vi "FPGAMain.vi"() -> ()   [LabVIEW 2022 SP3]
uses:
  <vilib>/rvi/Emulation/niFpgaGetClockAttributes.vi
  <vilib>/rvi/Emulation/niFpgaSctlEmulationGetInTimedLoop.vi
  <vilib>/rvi/Emulation/niFpgaEmulationReportErrorSimple.vi
  <vilib>/rvi/interface/RandomDataEmulation/niFpgaRandomDataHandleErrors.vi
  <vilib>/rvi/Emulation/niFpgaEmulationIsFPGAContextNoSignature.vi
  <vilib>/rvi/DataTransferAndStorage/Container/Common/niFpgaContainerGetUniqueNameForEmu.vi
  <vilib>/rvi/Memory/Memory_Emulation/niFpgaMemoryEmulationCacheClearOnFirstRun.vi
  <vilib>/rvi/Memory/Memory_Emulation/nirvimemoryEmulationManagerCache_MakeExclusive.vi
  <vilib>/rvi/Memory/Memory_Emulation/niFpgaMemoryEmulationValidateCache.vi
  <vilib>/rvi/Memory/Memory_Emulation/nirvimemoryEmulationManagerCache_InsertValue.vi
  <vilib>/Utility/error.llb/Clear Errors.vi
  <vilib>/rvi/Memory/Memory_Emulation/nirvimemoryEmulationManagerCache_ReleaseExclusive.vi
  <vilib>/rvi/Memory/Memory_Emulation/nirvimemoryEmulationManagerCache_GetValue.vi
  <vilib>/rvi/Memory/Memory_Emulation/nirvimemoryEmulationManagerCache_SetValue.vi
  <vilib>/rvi/Emulation/niFpgaProcessEmulError.vi
  <vilib>/rvi/DataTransferAndStorage/Container/Common/niFpgaContainerExecOnDevCompGetState.vi
  <vilib>/rvi/errors/niFpgaSetErrorForExecOnDevCompSimple.vi
  <vilib>/rvi/eio/common/nirviEmuReportErrorAndStop.vi
  <vilib>/rvi/FIFO/Fifo_Resource/nirvififoEmulationSetSize.vi
  <vilib>/rvi/FIFO/Fifo_Resource/nirviFifoEmulationQueueMgr.vi
  <instcachedir>/0/nirviFifoEmulationQueueMgr_E5CAEC123FF24DC58D834DCA3CDAA9B5.lvgen/nirviFifoEmulationQueueMgr_E5CAEC123FF24DC58D834DCA3CDAA9B5_005.vi
  <vilib>/rvi/FIFO/Fifo_Resource/nirvififoEmulationDetermineInputValidOut.vi
  <vilib>/rvi/FIFO/Fifo_Resource/nirvififoEmulationCreateLock.vi
  <vilib>/rvi/FIFO/Fifo_Resource/nirvififoEmulationObtainLock.vi
  <vilib>/rvi/FIFO/Fifo_Resource/nirvififoEmulationReleaseLock.vi
  <vilib>/rvi/occurrence/nirviWaitOnOccurrenceBase.vi
  <vilib>/rvi/errors/nirviReportUnexpectedCaseInternalError.vi
  <vilib>/rvi/errors/nirviReportUnexpectedCaseInternalError (U32).vi
  <vilib>/rvi/Emulation/niFpgaCriticalErrorInLSC.vi
  <vilib>/rvi/eio/common/nirviEmuTemplateMethod_errors.vi
  <vilib>/rvi/DataTransferAndStorage/Container/XNode/niFpgaContainer.xnode
  <vilib>/rvi/interface/RandomDataEmulation/nirviRandomDataFpgaReadWriteTemplate.vi
  <vilib>/rvi/DataTransferAndStorage/Register/Emulation/niFpgaRegisterEmulation.vi
  <vilib>/rvi/FIFO/Fifo_Resource/niFpgaFifoEmulationRefIn.vi
  <vilib>/eio/EIONode/EIONode.xnode
panel:
  out "Control Signals":bool[](array[boolean])
  out "Tick Count(uSec)":u16
  out "Mod1/AI0":fxp<+/-,26,5>
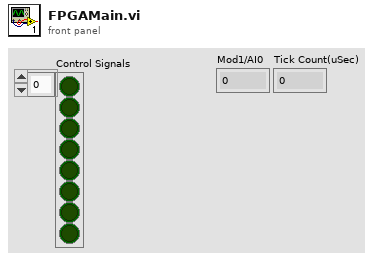
[diagram p1: front panel]
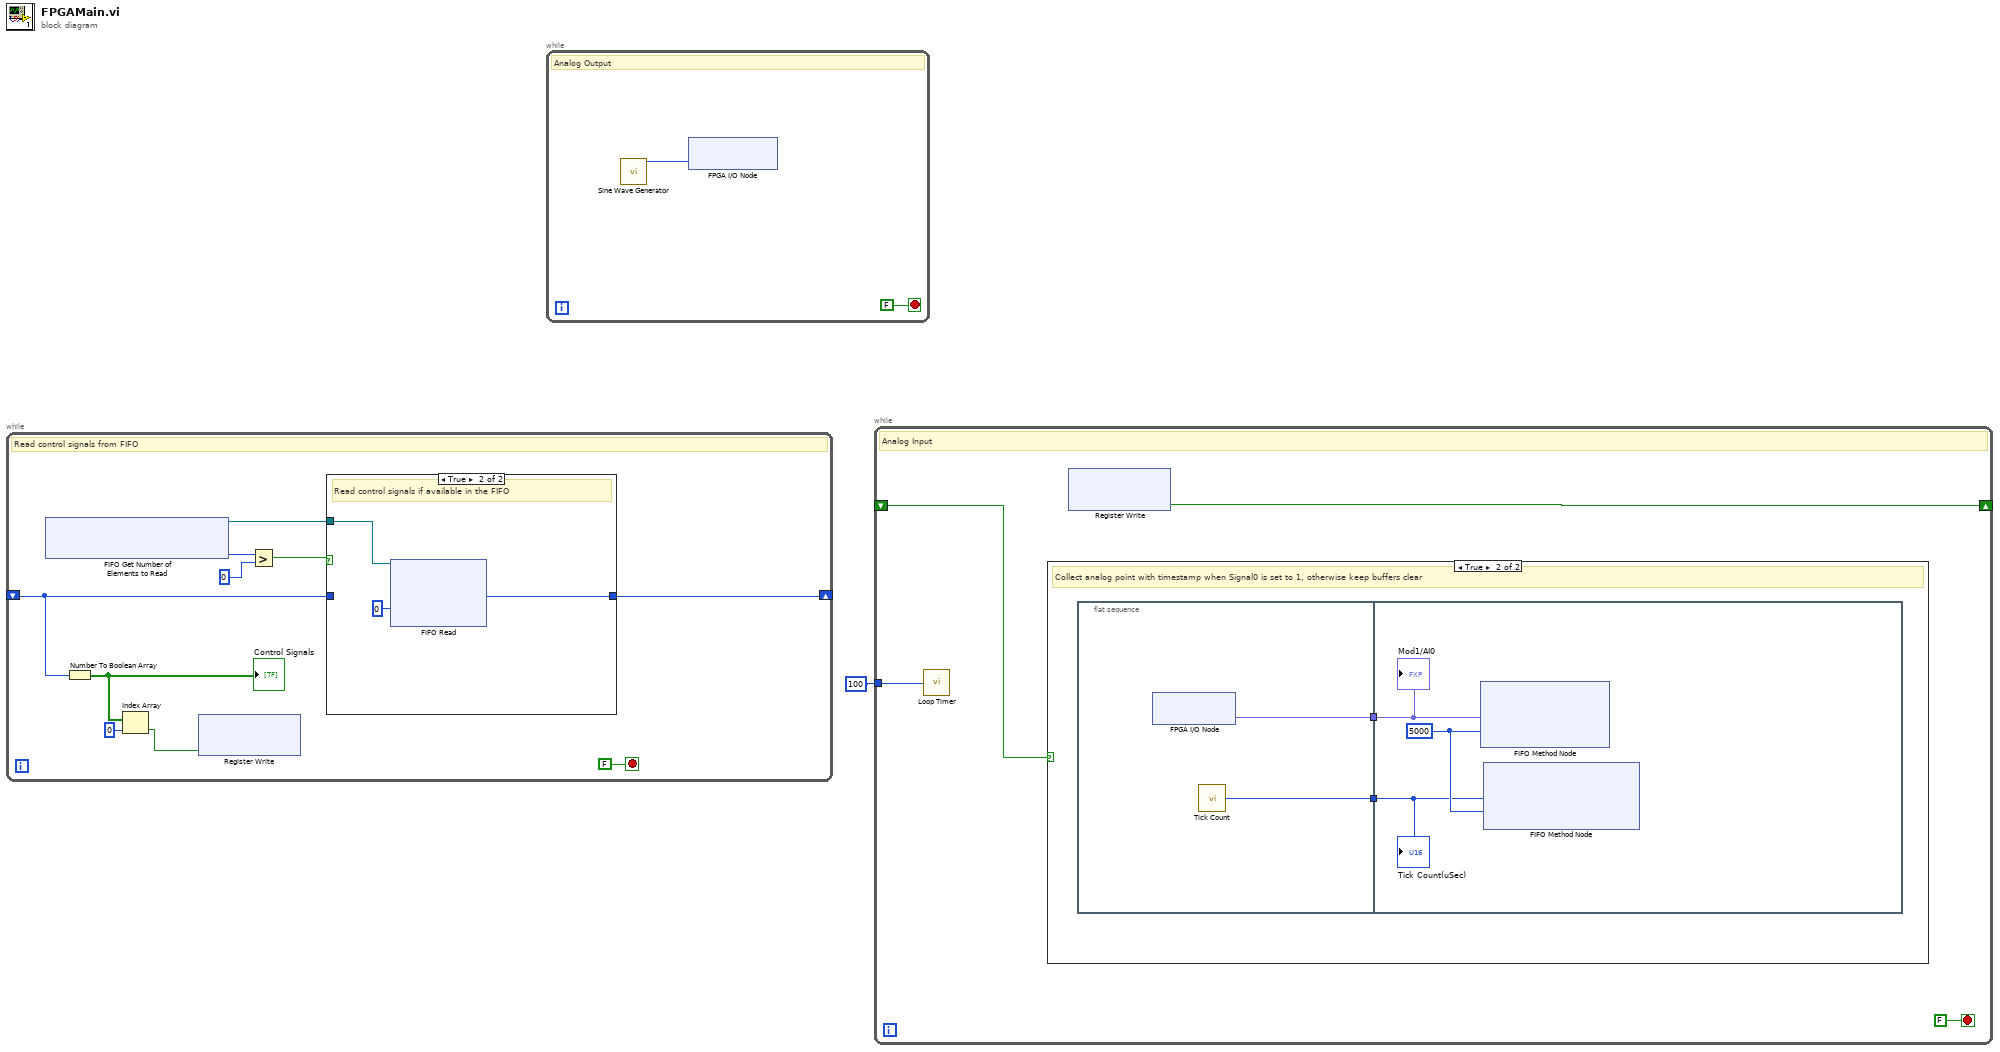
[diagram p0: block diagram]
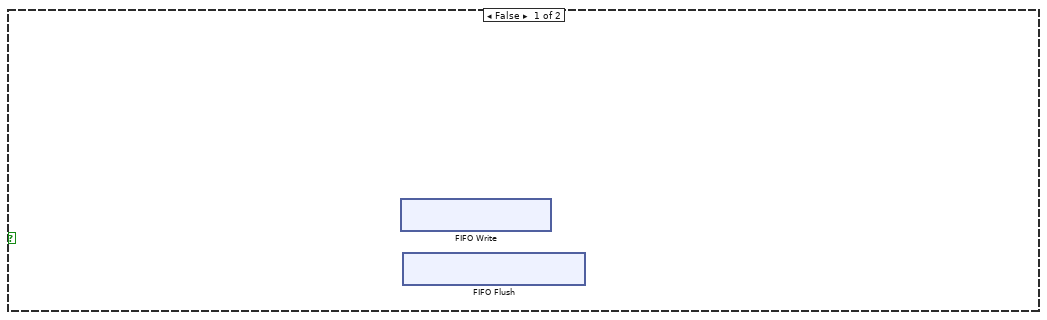
[diagram p2: hidden frame]
diagram:
  n1 = while {
    shift-right: [w5] -> _
    shift-left: _ -> [w6]
    stop <- FALSE stop-if-true
    # "Read control signals from FIFO"
    n2 = xnode "FIFO Get Number of Elements to Read"() -> ("Number of Elements to Read"=w10:u32, "FIFO Out"=w8:refnum<k21>)  [unwired: 1 in]
    n3 = Number To Boolean Array(number=w6) -> (Boolean array=w4:bool[])
    "Control Signals" <- w4
    n4 = Index Array(array=w4, index=0) -> (element=w3:bool)
    n5 = xnode "Register Write"("Data"=w3) -> ()  [unwired: 1 in, 1 out]
    n6 = Greater?(x=w10, y=u32 0) -> (0:w7:bool)
    n7 = case shown="True" w7 {
      tunnel: w8 -> [_ w15]
      tunnel: [w12 w13] -> w5
      tunnel: w6 -> [w12 _]
      frame False {
      }
      frame True {
        # "Read control signals if available in the FIFO"
        n8 = xnode "FIFO Read"("Timeout"=0, "FIFO In"=w15) -> ("Element"=w13:u8)  [unwired: 2 out]
      }
    }
  }
  n9 = while {
    stop <- FALSE stop-if-true
    # "Analog Output"
    n10 = call "Sine Wave Generator"() -> ("sine out"=w16:i16)  [unwired: 15 in]
    n11 = xnode "FPGA I/O Node"("Mod2/AO0"=w16) -> ()  [unwired: 1 in, 1 out]
  }
  n12 = while {
    tunnel: u32 100 ("Count(uSec)") -> [w20]
    shift-right: [w19] -> _
    shift-left: _ -> [w18]
    stop <- FALSE stop-if-true
    # "Analog Input"
    n13 = call "Loop Timer"("Count(Ticks)"=w20) -> ()  [unwired: 1 out]
    n14 = case shown="True" w18 {
      frame False {
        n15 = xnode "FIFO Write"() -> ()  [unwired: 1 in, 1 out]
        n16 = xnode "FIFO Flush"() -> ()  [unwired: 1 in, 1 out]
      }
      frame True {
        # "Collect analog point with timestamp when Signal0 is set to 1, otherwise keep buffers clear"
        n17 = flat-sequence {
          tunnel: [w25] -> w23
          tunnel: [w24] -> w22
          tunnel: w23 -> [w27]
          tunnel: w22 -> [w26]
          frame #0 {
            n18 = xnode "FPGA I/O Node"() -> ("Mod1/AI0"=w24:fxp<+/-,26,5>)  [unwired: 1 in, 1 out]
            n19 = call "Tick Count"() -> ("Tick Count(uSec)"=w25:u16)
          }
          frame #1 {
            w28 = 5000 ("Timeout")
            n20 = xnode ("FIFO Method Node")("Element"=w26, "Timeout"=w28) -> ()  [unwired: 1 in, 2 out]
            n21 = xnode ("FIFO Method Node")("Element"=w27, "Timeout"=w28) -> ()  [unwired: 1 in, 2 out]
            "Mod1/AI0" <- w26
            "Tick Count(uSec)" <- w27
          }
        }
      }
    }
    n22 = xnode "Register Write"() -> ("Data"=w19:bool)  [unwired: 1 in, 1 out]
  }
